vi "GetAllFunctionsFromProject.vi"(8 "error in (no error)":errorcluster, 11 "Path":path) -> (0 "error out":errorcluster, 3 "MethodPaths":path[](array[path]))   [LabVIEW 2020]
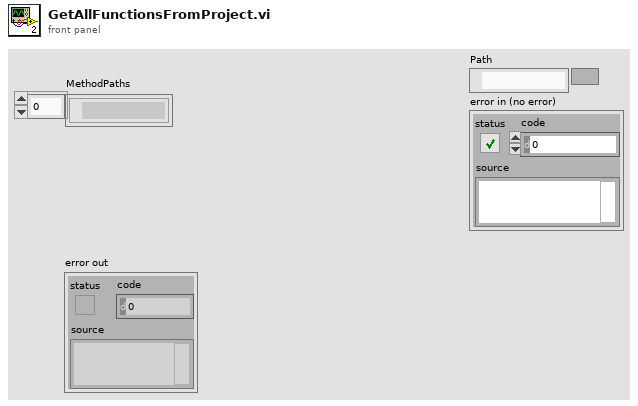
[diagram p1: front panel]
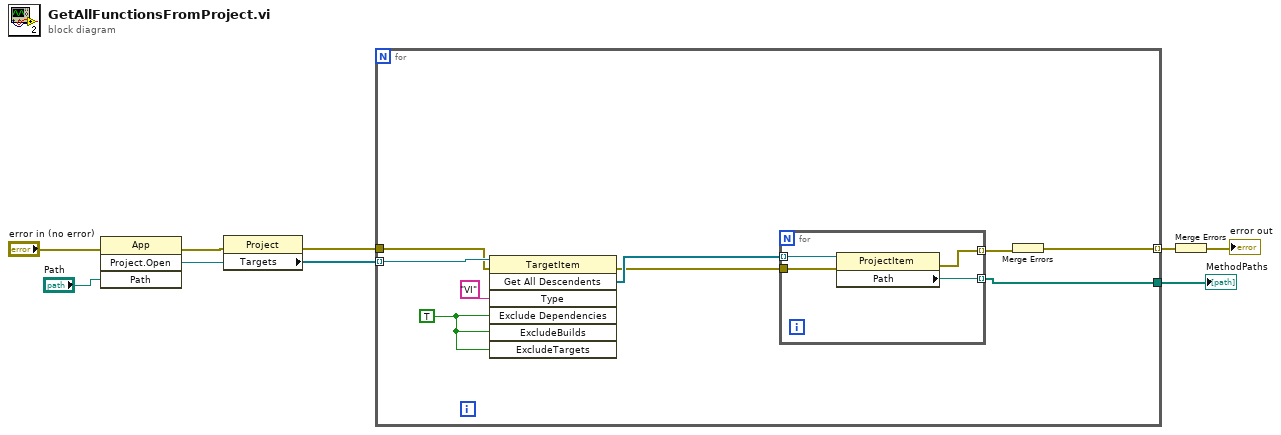
[diagram p0: block diagram]
diagram:
  n1 = invoke on="Invoke Node" class="App" method="Project.Open"(error in="error in (no error)", "Path"="Path") -> (error out=w8:errorcluster, "Project:Open"=w9:refnum<vi>)  [unwired: 2 in, 2 out]
  n2 = property on="Property Node" class="Project"(reference=w9, error in=w8) -> (error out=w6:errorcluster, "Targets"=w7:refnum<vi>[])  [unwired: 1 out]
  n3 = for {
    tunnel: w7 -> [w17] mode=indexing
    tunnel: w6 -> [w16]
    tunnel: [w15] -> w3
    tunnel: [w10] -> w5 mode=indexing
    w11 = TRUE ("ExcludeDependencies")
    n4 = invoke on="Invoke Node" class="TargetItem" method="Get All Descendents"(reference=w17, error in=w16, "Type"="VI", "Exclude Dependencies"=w11, "ExcludeBuilds"=w11, "ExcludeTargets"=w11) -> (error out=w13:errorcluster, "All Descendents"=w14:refnum<vi>[])  [unwired: 1 in, 5 out]
    n5 = for {
      tunnel: [w22] -> w15 mode=indexing
      tunnel: [w21] -> w18 mode=indexing
      tunnel: w14 -> [w20] mode=indexing
      tunnel: w13 -> [w19]
      n6 = property on="Property Node" class="ProjectItem"(reference=w20, error in=w19) -> (error out=w21:errorcluster, "Path"=w22:path)  [unwired: 1 out]
    }
    n7 = Merge Errors(w18) -> (w10:errorcluster)
  }
  "MethodPaths" <- w3
  n8 = Merge Errors(w5) -> (→"error out":errorcluster)
